vi "dfd_Cosine Modulated Analysis Bank with State (Array).vi"(6 "state in":cluster{"state ":dbl[]}[](array[cluster]), 7 "init?":bool, 8 "error in (no error)":errorcluster, 10 "bank in":T1={"mBank_Filters"=[], " mBank_#Bands"=2, "mBank_ProcMethod"=enum."General", "mBank_Coeffs"=[], "mBank_Gain"=1.0, "mBank_Type"=0} {"mBank_Type" items=["Uniform", "Non-Uniform"]; "mBank_Filters"."mMRate_SumWl" min=1 max=32 step=1; "mBank_Filters"."mMRate_InputIwl" min=1 max=32 step=1; "mBank_Filters"."mMRate_GainWl" min=1 max=32 step=1; "mBank_Filters"."mMRate_OutputWl" min=1 max=32 step=1; "mBank_Filters"."mMRate_InputWl" min=1 max=32 step=1; "mBank_Filters"."mMRate_CoefWl" min=1 max=32 step=1; "mBank_Filters"."mMRate_Mode" items=["Default"=-1, "No Rate Change"=0, "Interpolation"=1, "Decimation"=2, "Interpolated"=3, "Rational"=4]}, 11 "x":dbl[](array[numeric]) format="%.2f") -> (0 "error out":errorcluster, 3 "y":dbl[][](array[numeric]), 4 "state out":cluster{"state ":dbl[]}[](array[cluster]))   [LabVIEW 2017, in "NI_DigFilter_FilterBank.lvlib"]
uses:
  <vilib>/addons/Digital Filter Design/NI_DigFilter_FilterBank.lvlib
  <vilib>/addons/Digital Filter Design/FilterBank.llb/Object/DFD Bank Obj.ctl
  <vilib>/addons/Digital Filter Design/_Objects.llb/DFD Multirate Filter Obj.ctl
  <vilib>/addons/Digital Filter Design/_Objects.llb/DFD Multirate Mode.ctl
  <vilib>/addons/Digital Filter Design/_Objects.llb/DFD Coef Norm Type.ctl
  <vilib>/addons/Digital Filter Design/_Objects.llb/DFD Round-off Mode.ctl
  <vilib>/addons/Digital Filter Design/_Objects.llb/DFD FXP MRate Multiply Mode.ctl
  <vilib>/addons/Digital Filter Design/FilterBank.llb/Object/DFD Filter Bank Processing Method.ctl
  <vilib>/addons/Digital Filter Design/FilterBank.llb/Object/DFD Filter Bank Type.ctl
  <vilib>/addons/Digital Filter Design/_Misc.llb/dfd_Error Cluster From Error Code (Scalar).vi
  <vilib>/addons/Digital Filter Design/NI_DigFilterLicensed.lvlib
  <resource>/LVDFD.dll
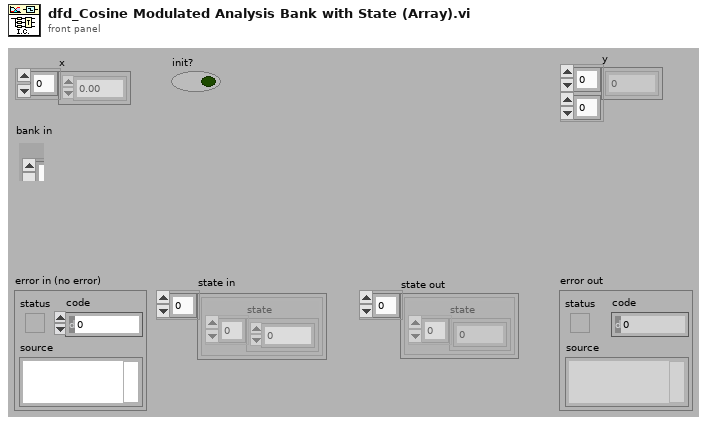
[diagram p1: front panel]
types:
  T1 = typedef "NI_DigFilter_FilterBank.lvlib/DFD Bank Obj.ctl" = cluster{"mBank_Filters":T2[], " mBank_#Bands":i32, "mBank_ProcMethod":T7, "mBank_Coeffs":dbl[], "mBank_Gain":dbl, "mBank_Type":T8}
  T2 = typedef "NI_DigFilterLicensed.lvlib/DFD Multirate Filter Obj.ctl" = cluster{"mMRate_Structure":enum16{"CIC", "FIR", "IIR", "Lattice"}, "mMRate_Mode":T3, "mMRate_Factor":i32, "mMRate_FIRParams":cluster{"mMRate_FIR_H":dbl[], "mMRate_FIR_IsNyquist?":bool, "mMRate_FIR_IsSymmetric?":bool}, "mMRate_CICParams":cluster{"mMRate_CIC_#Stage":i32, "mMRate_CIC_Lag":i32, "mMRate_CIC_Type":enum16{"Lowpass", "Highpass"}}, "mMRate_Order":i32, "mMRate_Version":string, "mMRate_Comments":string, "mMRate_RationalFactor":cluster{"mMRate_L":i32, "mMRate_M":i32}, "mMRate_Fs":dbl, "mMRate_Quantized?":bool, "mMRate_QFilterGain":dbl, "mMRate_CoefWl":i16, "mMRate_Scaling":cluster{"mMRate_ScaleByPowerOf2?":bool, "mMRate_ScaleType":T4}, "mMRate_InputWl":i16, "mMRate_OutputWl":i16, "mMRate_OutputMode":T5, "mMRate_MultMode":T6, "mMRate_BitPruning":bool, "mMRate_GainWl":i16, "mMRate_OutputFwl":i16, "mMRate_SumIwl":i16, "mMRate_InputIwl ":i16, "mMRate_SumWl":i16, "mMRate_CoefIwl":i16}
  T3 = typedef "NI_DigFilterLicensed.lvlib/DFD Multirate Mode.ctl" = i16
  T4 = typedef "NI_DigFilterLicensed.lvlib/DFD Coef Norm Type.ctl" = enum16{"No Norm", "Time Domain 1-Norm", "Time Domain 2-Norm", "Time Domain Inf-Norm"}
  T5 = typedef "NI_DigFilterLicensed.lvlib/DFD Round-off Mode.ctl" = enum16{"Nearest", "Truncation"}
  T6 = typedef "NI_DigFilterLicensed.lvlib/DFD FXP MRate Multiply Mode.ctl" = enum16{"Truncated", "Full"}
  T7 = typedef "NI_DigFilter_FilterBank.lvlib/DFD Filter Bank Processing Method.ctl" = enum16{"General", "2-Band QMF Lattice", "Cosine-Modulated"}
  T8 = typedef "NI_DigFilter_FilterBank.lvlib/DFD Filter Bank Type.ctl" = u16
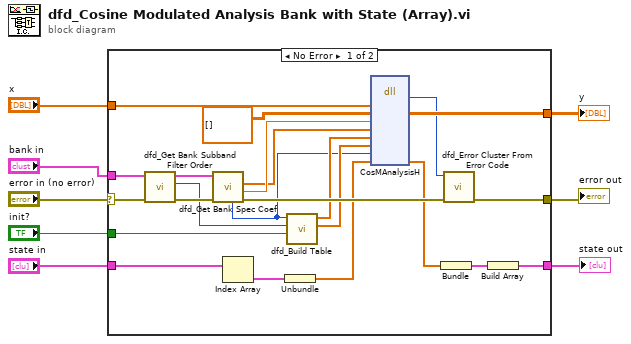
[diagram p0: block diagram]
diagram:
  n1 = case shown="No Error" "error in (no error)" {
    selector: "error in (no error)" -> [w27 w32]
    tunnel: "x" -> [w29 _]
    tunnel: [w31 _] -> w8
    tunnel: [w30 w32] -> w7
    tunnel: [w10 _] -> w5
    tunnel: "state in" -> [w28 _]
    tunnel: "bank in" -> [w26 _]
    tunnel: "init?" -> [w25 _]
    frame No Error {
      n2 = call <vilib>:"dfd_Get Bank Subband Filter Order.vi"("error in (no error)"=w27, "bank in"=w26) -> ("error out"=w14:errorcluster, "order"=w12:i32, "bank out"=w13:T1)  [unwired: 7 in]
      n3 = call <vilib>:"dfd_Get Bank Spec Coef.vi"("error in (no error)"=w14, "bank in"=w13) -> ("error out"=w23:errorcluster, "gain"=w24:dbl, "coefficients"=w18:dbl[], "number of bands"=w15:i32)  [unwired: 4 in, 2 out]
      n4 = Index Array(array=w28) -> (element=w22:cluster{"state ":dbl[]})  [unwired: 1 in]
      n5 = Unbundle(w22) -> ("state"=w20:dbl[])
      n6 = call <vilib>:"dfd_Build Table.vi"("init?"=w25, "order"=w12, "channel"=w15) -> ("table"=w16:dbl[], "sincostable"=w17:dbl[])  [unwired: 7 in]
      n7 = dll-call lib="C:/Program Files/National Instruments/LabVIEW 2017/resource/LVDFD.*" fn="CosMAnalysisH"("input"=w29, "output"=dbl[][] [], "gain"=w24, "coeff"=w18, "sinecos_table"=w17, "table"=w16, "bandH"=w15, "foreStates"=w20) -> ("return type"=w21:i32, "output"=w31:dbl[][], "foreStates"=w19:dbl[])  [unwired: 9 in, 2 out]
      n8 = Bundle("foreStates"=w19) -> (w9:cluster{"foreStates":dbl[]})  [unwired: 1 in]
      n9 = call-poly <vilib>:"dfd_Error Cluster From Error Code.vi"("error in (no error)"=w23, "error code (0)"=w21) -> ("error out"=w30:errorcluster)  [unwired: 9 in]
      n10 = Build Array(w9) -> (w10:cluster{"foreStates":dbl[]}[])
    }
    frame Error {
    }
  }
  "y" <- w8
  "error out" <- w7
  "state out" <- w5
